vi "Read XML Handler.lvclass.vi"(11 "Measurements in":refnum<class "Measurement.lvclass">) -> (2 "XML Handler.lvclass":refnum<class "XML Handler.lvclass">, 3 "Measurements out":refnum<class "Measurement.lvclass">)   [LabVIEW 2020, in "Measurement.lvclass"]
uses:
  Measurement.lvclass
  XML Handler/XML Handler.lvclass
  Measurement.lvclass/Measurement.ctl
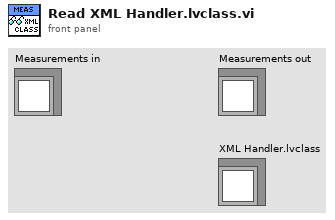
[diagram p1: front panel]
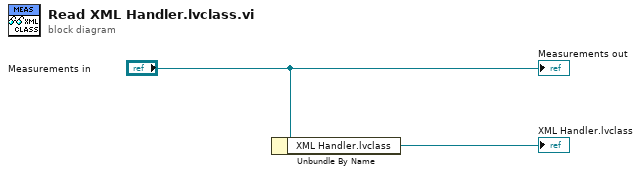
[diagram p0: block diagram]
diagram:
  n1 = Unbundle By Name("Measurements in") -> ("XML Handler.lvclass"=→"XML Handler.lvclass":refnum<class "XML Handler.lvclass">)
  "Measurements out" <- "Measurements in"
